vi "disable_all_channels_set_one.vi"() -> ()   [LabVIEW 2009]
panel:
  in  "Channel":u32
  in  "Clip_sel_b":u32
  in  "Ib_clipVb":u32
  in  "Att gain":u32=4095
  in  "error in":errorcluster
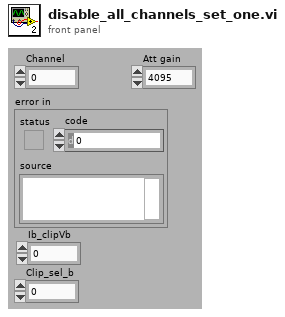
[diagram p1: front panel]
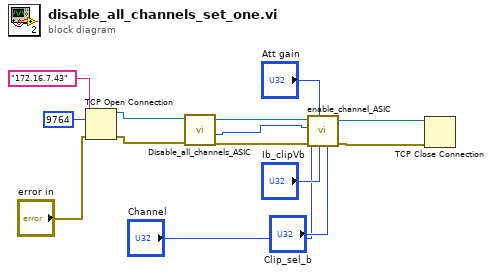
[diagram p0: block diagram]
diagram:
  n1 = TCP Open Connection(address="172.16.7.43", remote port or service name=u16 9764, error in (no error)="error in") -> (connection ID=w9:refnum<k5>, error out=w11:errorcluster)  [unwired: 2 in]
  n2 = call "Disable_all_channels_ASIC.vi"("error in"=w11, "connection ID"=w9) -> ("error out"=w13:errorcluster, "id_out"=w5:i32, "connection ID out"=w14:refnum<k5>)  [unwired: 7 in]
  n3 = call "enable_channel_ASIC.vi"("Clip_sel_b"="Clip_sel_b", "Ib_clipVb"="Ib_clipVb", "Att gain"="Att gain", "error in"=w13, "Channel"="Channel", "id_in"=w5, "connection ID"=w14) -> ("error out"=w7:errorcluster, "connection ID out"=w6:refnum<k5>)  [unwired: 2 in, 1 out]
  n4 = TCP Close Connection(connection ID=w6, error in (no error)=w7) -> ()  [unwired: 1 in, 2 out]
